vi "Stop Core.vi"(10 "final error code":i32 caption="最终错误代码", 11 "MiddleSlaveActor in":refnum<class "MiddleSlaveActor.lvclass"> caption="操作者输入") -> (3 "MiddleSlaveActor out":refnum<class "MiddleSlaveActor.lvclass"> caption="操作者输出")   [LabVIEW 2014, in "UnitTest.lvlib" / "MiddleSlaveActor.lvclass"]
doc: "(<B>文件名</B>：Actor Framework.lvlib:Actor.lvclass:Stop Core.vi)\n\n定义停止前操作者的动作。使用<B>最终错误代码</B>输入判断操作者是否在出错时关闭。\n\n默认情况下，该方法不执行任何动作。子孙类重写该方法，定义出错时的操作，例如，关闭操作者核心方法初始的进程。"
uses:
  MiddleSlaveActor.lvclass
  <vilib>/ActorFramework/Actor/Actor.lvclass
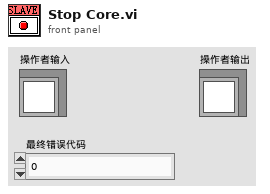
[diagram p1: front panel]
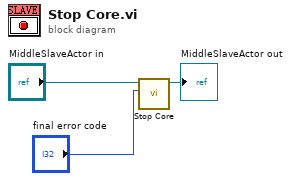
[diagram p0: block diagram]
diagram:
  n1 = call-parent "Stop Core.vi"("final error code"="final error code", "Actor in"="MiddleSlaveActor in") -> ("Actor out"=→"MiddleSlaveActor out":refnum<class "MiddleSlaveActor.lvclass">)  [unwired: 9 in]
